vi "Picture Dial.vi"() -> ()   [LabVIEW 2023]
doc: "Combines a picture control with a dial to have a picture within a dial. The picture control is grouped and locked to the dial along with a decoration to cover the corners of the picture control.\n\n*Notice the use of a stored pixmap image so the image is saved with the VI itself."
uses:
  Rotate.llb/rotate 24bit.vi
panel:
  in  "stop":bool
  in  "Stored Pixmap Image":u32[][](array[numeric])=array212x212[44944 elements] format="%.0x"
  in  "Dial":dbl(knob)=4.820308593039098 scale=0.0..10.0
  out "Picture":picture
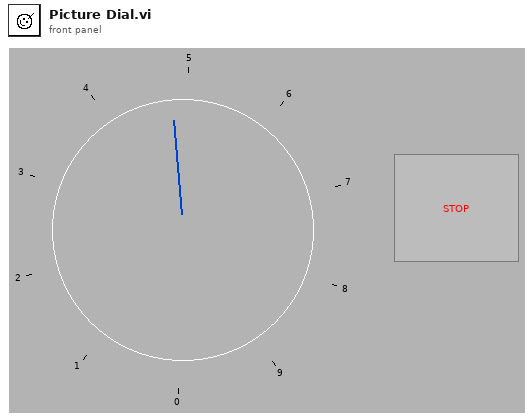
[diagram p1: front panel]
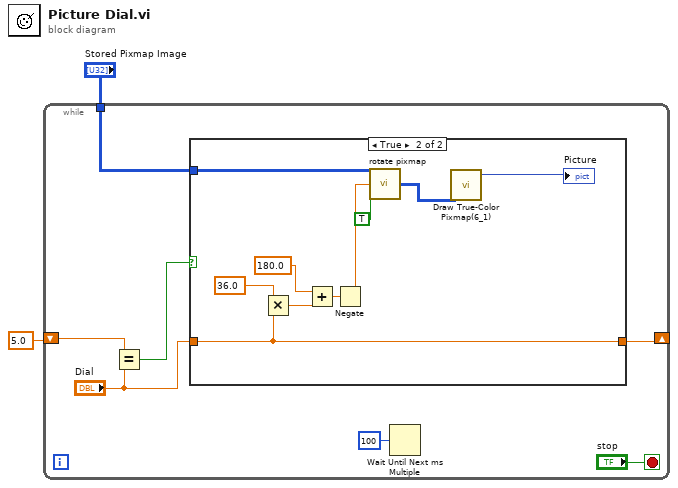
[diagram p0: block diagram]
diagram:
  n1 = while {
    shift-right: [w5] -> _
    shift-left: 5.0 -> [w9]
    tunnel: "Stored Pixmap Image" -> [w7]
    stop <- "stop" stop-if-true
    n2 = Equal?(x=w9, y="Dial") -> (x = y?=w8:bool)
    n3 = case shown="True" w8 {
      tunnel: w7 -> [_ w17]
      tunnel: "Dial" -> [w10 w13]
      tunnel: [w10 w13] -> w5
      frame False {
      }
      frame True {
        n4 = Multiply(x=36.0, y=w13) -> (x*y=w19:dbl)
        n5 = Add(x=180.0, y=w19) -> (x+y=w12:dbl)
        n6 = Negate(x=w12) -> (-x=w11:dbl)
        n7 = call-poly "rotate pixmap.vi"("Maintain Center Position?"=TRUE, "Rotation Angle (degrees)"=w11, "Pixmap"=w17) -> ("Rotated Pixmap"=w15:u32[][])  [unwired: 1 in]
        n8 = call <vilib>:"Draw True-Color Pixmap(6_1).vi"("data (RGB format)"=w15) -> ("new picture"=→"Picture":picture)  [unwired: 8 in]
      }
    }
    n9 = Wait Until Next ms Multiple(millisecond multiple=u32 100) -> ()  [unwired: 1 out]
  }
